vi "gfitsio-not-a-refnum.vi"() -> (0 "invalid gfits refnum":T1)   [LabVIEW 2022 SP3, in "gfitsio.lvlib"]
uses:
  gfitsio.lvlib
  gfitsio-refnum.ctl
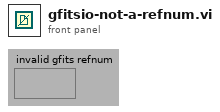
[diagram p1: front panel]
types:
  T1 = typedef "gfitsio.lvlib/gfitsio-refnum.ctl" = refnum<k1>
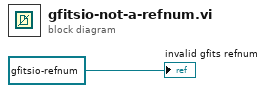
[diagram p0: block diagram]
diagram:
  w1 = T1 refnum items=["GFITSIO"] ("GFITSIO File Refnum")
  "invalid gfits refnum" <- w1
